vi "M05 Smart Grid.vi"(9 "Target angle":sgl, 11 "EV3 in":T1) -> (3 "EV3 out":T1)   [LabVIEW 2016]
uses:
  <vilib>/NXT/Subs/LVHSConnector.ctl
  <vilib>/NXT/LegoClasses/BrickReference/BrickReference.lvclass
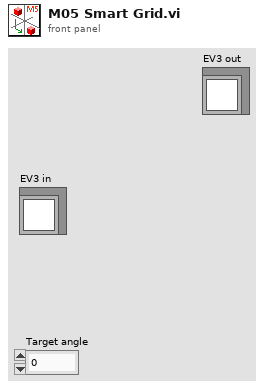
[diagram p1: front panel]
types:
  T1 = typedef "LVHSConnector.ctl" = refnum<class "BrickReference.lvclass">
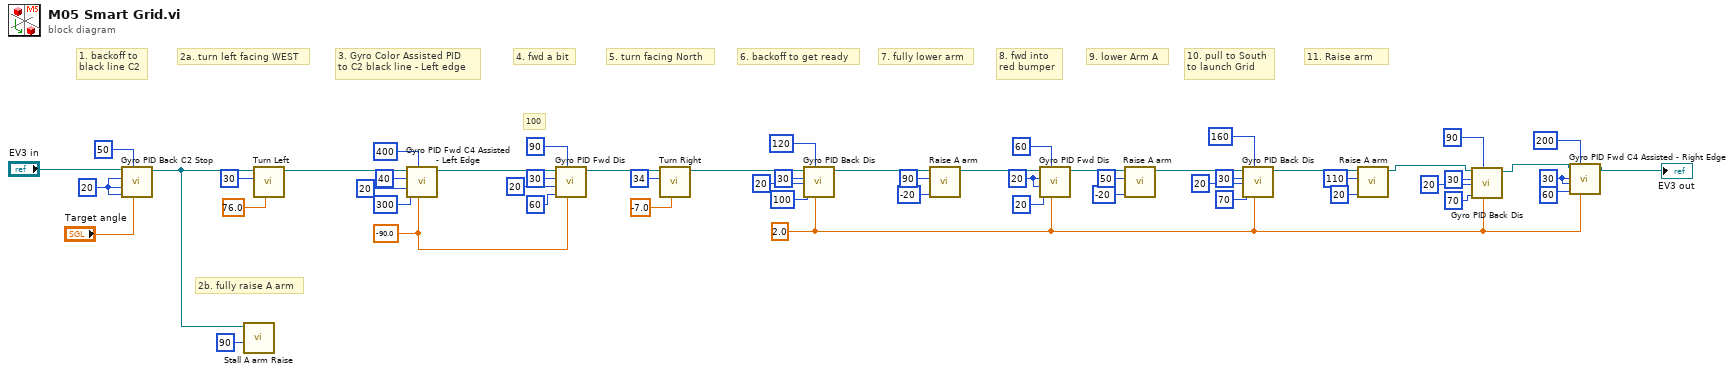
[diagram p0: block diagram]
diagram:
  w9 = 30 ("Max. speed")
  w12 = 20 ("Max. speed")
  w2 = sgl 2.0 ("Target angle")
  w33 = 20 ("Max. speed")
  w45 = sgl -90.0 ("Target angle")
  # "100"
  # "11. Raise arm"
  # "9. lower Arm A"
  # "8. fwd into\nred bumper"
  # "7. fully lower arm"
  # "6. backoff to get ready"
  # "2b. fully raise A arm"
  # "1. backoff to\nblack line C2"
  # "10. pull to South\nto launch Grid"
  # "5. turn facing North"
  # "4. fwd a bit"
  # "3. Gyro Color Assisted PID\nto C2 black line - Left edge"
  # "2a. turn left facing WEST"
  n1 = call "Gyro PID Back C2 Stop.vi"("Target angle"="Target angle", "Threshold to Color"=50, "Threshold to slow"=w33, "Min. speed"=w33, "Max. speed"=w33, "EV3 in"="EV3 in") -> ("EV3 out"=w13:T1)  [unwired: 5 in]
  n2 = call "Stall A arm Raise.vi"("Power"=i8 90, "NXT/EV3"=w13) -> ()  [unwired: 9 in, 1 out]
  n3 = call "Turn Left.vi"("Turning angle"=sgl 76.0, "Motor B (right)"=i8 30, "EV3 in"=w13) -> ("EV3 out"=w37:T1)  [unwired: 8 in]
  n4 = call "Gyro PID Fwd C4 Assisted - Left Edge.vi"("Target angle"=w45, "Threshold to Color"=400, "Threshold to slow"=300, "Min. speed"=20, "Max. speed"=40, "EV3 in"=w37) -> ("EV3 out"=w50:T1)  [unwired: 5 in]
  n5 = call "Gyro PID Fwd Dis.vi"("Target angle"=w45, "Threshold to stop"=90, "Threshold to slow"=60, "Min. speed"=20, "Max. speed"=30, "EV3 in"=w50) -> ("EV3 out"=w44:T1)  [unwired: 5 in]
  n6 = call "Turn Right.vi"("Turning angle"=sgl -7.0, "Motor B (right)"=i8 34, "EV3 in"=w44) -> ("EV3 out"=w28:T1)  [unwired: 8 in]
  n7 = call "Gyro PID Back Dis.vi"("Target angle"=w2, "Threshold to stop"=120, "Threshold to slow"=100, "Min. speed"=20, "Max. speed"=30, "EV3 in"=w28) -> ("EV3 out"=w27:T1)  [unwired: 5 in]
  n8 = call "Raise A arm.vi"("Power"=i8 -20, "Rotation"=90, "EV3 in"=w27) -> ("EV3 out"=w24:T1)  [unwired: 8 in]
  n9 = call "Gyro PID Fwd Dis.vi"("Target angle"=w2, "Threshold to stop"=60, "Threshold to slow"=20, "Min. speed"=w12, "Max. speed"=w12, "EV3 in"=w24) -> ("EV3 out"=w23:T1)  [unwired: 5 in]
  n10 = call "Raise A arm.vi"("Power"=i8 -20, "Rotation"=50, "EV3 in"=w23) -> ("EV3 out"=w22:T1)  [unwired: 8 in]
  n11 = call "Gyro PID Back Dis.vi"("Target angle"=w2, "Threshold to stop"=160, "Threshold to slow"=70, "Min. speed"=20, "Max. speed"=30, "EV3 in"=w22) -> ("EV3 out"=w16:T1)  [unwired: 5 in]
  n12 = call "Raise A arm.vi"("Power"=i8 20, "Rotation"=110, "EV3 in"=w16) -> ("EV3 out"=w4:T1)  [unwired: 8 in]
  n13 = call "Gyro PID Back Dis.vi"("Target angle"=w2, "Threshold to stop"=90, "Threshold to slow"=70, "Min. speed"=20, "Max. speed"=30, "EV3 in"=w4) -> ("EV3 out"=w3:T1)  [unwired: 5 in]
  n14 = call "Gyro PID Fwd C4 Assisted - Right Edge.vi"("Target angle"=w2, "Threshold to Color"=200, "Threshold to slow"=60, "Min. speed"=w9, "Max. speed"=w9, "EV3 in"=w3) -> ("EV3 out"=→"EV3 out":T1)  [unwired: 5 in]
